vi "get_indices.vi"(8 "error in (no error)":errorcluster caption="entrée d'erreur (pas d'erreur)", 11 "SpectralBiclustering.lvclass":refnum<class "SpectralBiclustering.lvclass">) -> (0 "error out":errorcluster caption="sortie d'erreur", 2 "out":cluster{"row_ind":dbl, "col_ind":dbl}, 3 "SpectralBiclustering.lvclass 2":refnum<class "SpectralBiclustering.lvclass">)   [LabVIEW 2020, in "SpectralBiclustering.lvclass"]
doc: "Row and column indices of the i’th bicluster.\n\nOnly works if rows_ and columns_ attributes exist."
uses:
  SpectralBiclustering.lvclass
  C:/Users/cipop/TDF Dropbox/2_Technologies de France/1 - Services et Etudes/PLAIY/2 - DEV/PLAIYLAB/code/Python/Python.lvclass
  C:/Users/cipop/TDF Dropbox/2_Technologies de France/1 - Services et Etudes/PLAIY/2 - DEV/PLAIYLAB/code/Model/Model.lvclass
  SpectralBiclustering.lvclass/SpectralBiclustering.ctl
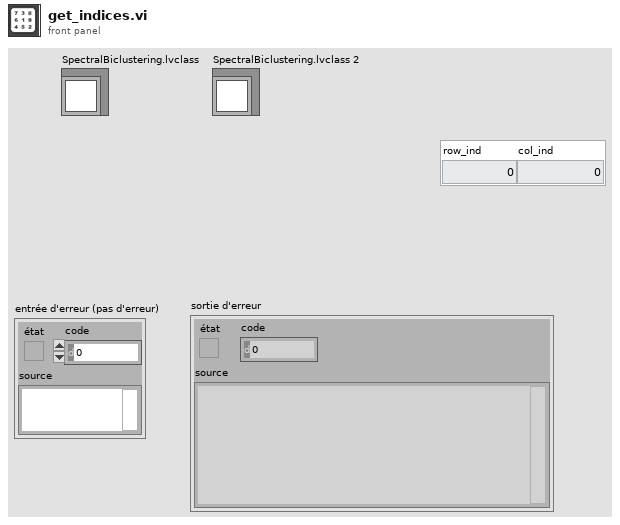
[diagram p1: front panel]
types:
  T1 = typedef "data.ctl" = cluster{"name":string, "X":dbl[][]}
  T2 = typedef "spectral_biclustering_data.ctl" = cluster{"i":dbl, "data":dbl[][]}
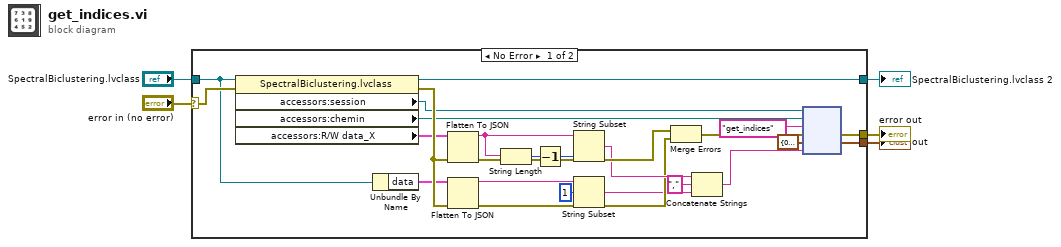
[diagram p0: block diagram]
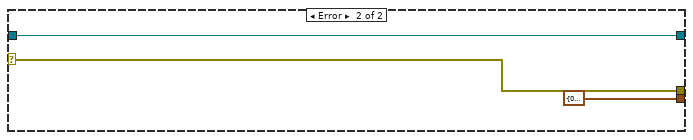
[diagram p2: hidden frame]
diagram:
  n1 = case shown="No Error" "error in (no error)" {
    selector: "error in (no error)" -> [w27 w32]
    tunnel: [w28 w32] -> w2
    tunnel: [w6 w31] -> w3
    tunnel: "SpectralBiclustering.lvclass" -> [w11 w31]
    tunnel: [w13 cluster{"row_ind":dbl, "col_ind":dbl} {"row_ind"=0.0, "col_ind"=0.0} ("out")] -> w1
    frame No Error {
      n2 = property class="SpectralBiclustering.lvclass"(reference=w11, error in=w27) -> (reference out=w6:refnum<class "SpectralBiclustering.lvclass">, error out=w18:errorcluster, "accessors:session"=w8:refnum<k35>, "accessors:chemin"=w7:path, "accessors:R/W data_X"=w12:T1)
      n3 = Unbundle By Name(w11) -> ("data"=w10:T2)
      n4 = Flatten To JSON(anything=w12, error in (no error)=w18) -> (JSON string=w24:string, 11:w21:errorcluster)  [unwired: 1 in]
      n5 = Flatten To JSON(anything=w10, error in (no error)=w18) -> (JSON string=w22:string, 11:w17:errorcluster)  [unwired: 1 in]
      n6 = String Length(string=w24) -> (length=w26:i32)
      n7 = Decrement(x=w26) -> (x-1=w25:i32)
      n8 = String Subset(string=w24, length (rest)=w25) -> (substring=w20:string)  [unwired: 1 in]
      n9 = String Subset(string=w22, offset (0)=1) -> (substring=w15:string)  [unwired: 1 in]
      n10 = Merge Errors(w21, w17) -> (w9:errorcluster)
      n11 = Concatenate Strings(w20, "," ("string"), w15) -> (w19:string)
      n12 = node(w8, w7, "get_indices" ("nom de la fonction"), w9, cluster{"row_ind":dbl, "col_ind":dbl} {"row_ind"=0.0, "col_ind"=0.0} ("out"), w19) -> (w28:errorcluster, w13:cluster{"row_ind":dbl, "col_ind":dbl})  [unwired: 1 in, 3 out]
    }
    frame Error {
    }
  }
  "error out" <- w2
  "SpectralBiclustering.lvclass 2" <- w3
  "out" <- w1
